vi "Autonomous.vi"() -> ()   [LabVIEW 2017]
doc: "This VI starts when autonomous period begins, and will automatically be terminated when it ends. You can carry out timed or sensor driven operations directly to I/O or to subsystems without needing to return to the caller."
uses:
  Shared/PathFileData.ctl
  Support Code/AutonomousRoutine.ctl
  b2a3c205-1cfd-49ae-9965-d89eaaa89800.vi
  <vilib>/Rock Robotics/WPI/Utilities/WPI_GetSetVariantRefNum.vi
  <vilib>/Rock Robotics/Network Tables/NT Read Boolean.vi
  <vilib>/Rock Robotics/Network Tables/NT Read Numeric Array.vi
  <vilib>/Rock Robotics/Network Tables/NT Read Number.vi
panel:
  out "PathData":T1
  out "File Path":string
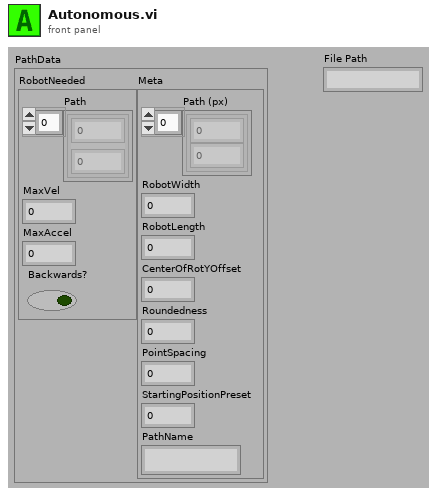
[diagram p1: front panel]
types:
  T1 = typedef "PathFileData.ctl" = cluster{"RobotNeeded":cluster{"Path":cluster{dbl, dbl}[], "MaxVel":dbl, "MaxAccel":dbl, "Backwards?":bool}, "Meta":cluster{"Path (px)":cluster{i32, i32}[], "RobotWidth":dbl, "RobotLength":dbl, "CenterOfRotYOffset":dbl, "Roundedness":dbl, "PointSpacing":dbl, "StartingPositionPreset":u32, "PathName":string}}
  T2 = typedef "AutonomousRoutine.ctl" = enum16{"Score Scale", "Score Switch"}
  T3 = typedef "WPI_JoystickDevRef.ctl" = cluster{"Device":T4}
  T4 = typedef "WPI_JoystickDeviceEnum.ctl" = enum16{"USB 0", "USB 1", "USB 2", "USB 3", "USB 4", "USB 5"}
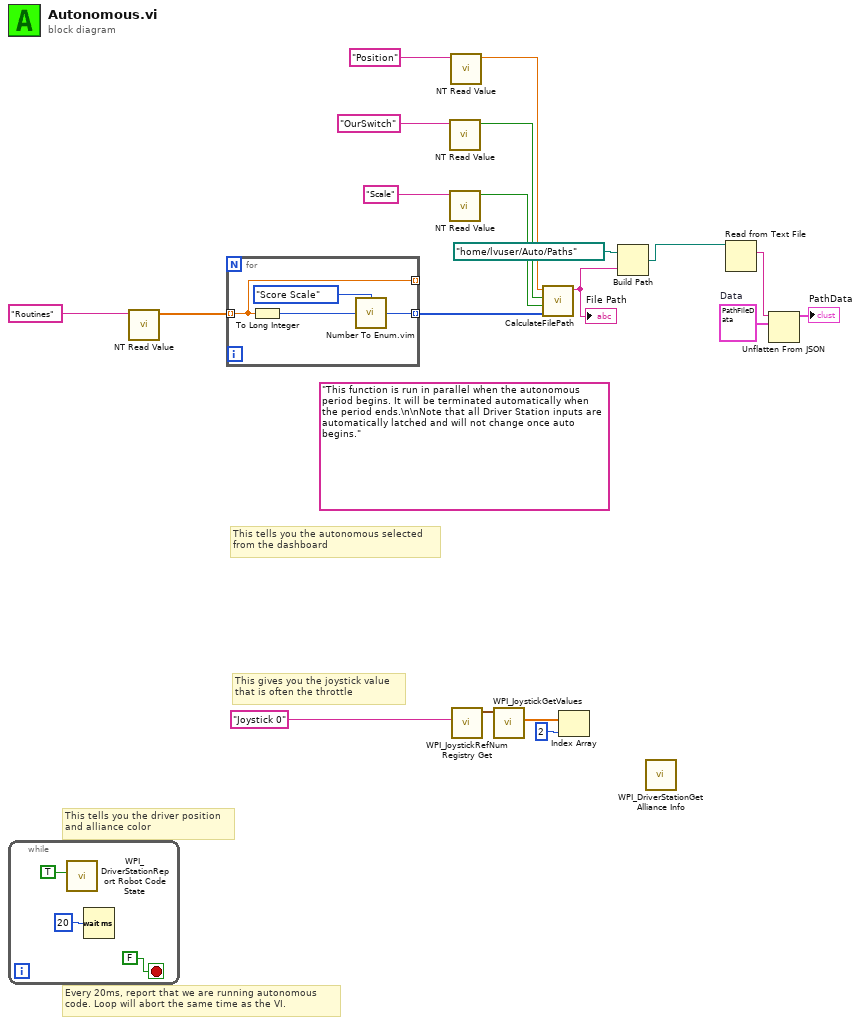
[diagram p0: block diagram]
diagram:
  w2 = T1 {"RobotNeeded"={"Path"=[], "MaxVel"=0.0, "MaxAccel"=0.0, "Backwards?"=FALSE}, "Meta"={"Path (px)"=[], "RobotWidth"=0.0, "RobotLength"=0.0, "CenterOfRotYOffset"=0.0, "Roundedness"=0.0, "PointSpacing"=0.0, "StartingPositionPreset"=0, "PathName"=""}}  # Data
  (unwired) "This function is run in parallel when the autonomous period begins. It will be terminated automatically when the period ends.\n\nNote that all Driver Station inputs are automatically latched and will not change once auto begins."
  # "This tells you the autonomous selected\nfrom the dashboard"
  # "Every 20ms, report that we are running autonomous\ncode. Loop will abort the same time as the VI."
  # "This gives you the joystick value\nthat is often the throttle"
  # "This tells you the driver position\nand alliance color"
  n1 = while {
    stop <- FALSE stop-if-true
    n2 = call <vilib>:"WPI_DriverStationReport Robot Code State.vi"("Autonomous"=TRUE) -> ()  [unwired: 10 in, 1 out]
    n3 = Wait (ms)(milliseconds to wait=u32 20) -> ()  [unwired: 1 out]
  }
  n4 = call-poly <vilib>:"NT Read Value.vi"("Name"="Routines") -> ("Numeric Array"=w11:dbl[])  [unwired: 9 in, 1 out]
  n5 = for {
    tunnel: w11 -> [w26] mode=indexing
    tunnel: [w26] -> _ mode=indexing
    tunnel: [w23] -> w7 mode=indexing
    n6 = To Long Integer(number=w26) -> (32bit integer=w25:i32)
    n7 = call "Number To Enum.vim"("number"=w25, "enum type"=AutonomousRoutine."Score Scale" ("LL")) -> ("number as enum"=w23:T2)
  }
  n8 = call-poly <vilib>:"NT Read Value.vi"("Name"="OurSwitch") -> ("Boolean"=w9:bool)  [unwired: 9 in, 1 out]
  n9 = call-poly <vilib>:"NT Read Value.vi"("Name"="Scale") -> ("Boolean"=w8:bool)  [unwired: 9 in, 1 out]
  n10 = call-poly <vilib>:"NT Read Value.vi"("Name"="Position") -> ("Numeric"=w10:dbl)  [unwired: 9 in, 1 out]
  n11 = call <vilib>:"WPI_JoystickRefNum Registry Get.vi"("refnum name"="Joystick 0") -> ("JoystickDevRef"=w18:T3)  [unwired: 1 in, 9 out]
  n12 = call <vilib>:"WPI_JoystickGetValues.vi"("JoystickDevRef"=w18) -> ("Axes"=w17:dbl[])  [unwired: 6 in, 4 out]
  n13 = call "CalculateFilePath.vi"("Routines"=w7, "Scale"=w8, "OurSwitch"=w9, "Position"=w10) -> ("File Name"=w6:string)  [unwired: 7 in]
  "File Path" <- w6
  n14 = Index Array(array=w17, index=2) -> ()  [unwired: 1 out]
  n15 = Build Path(base path=path "/home/lvuser/Auto/Paths", name or relative path=w6) -> (appended path=w4:path)
  n16 = call <vilib>:"WPI_DriverStationGet Alliance Info.vi"() -> ()  [unwired: 12 out]
  n17 = Read from Text File(file (use dialog)=w4) -> (text=w3:string)  [unwired: 3 in, 3 out]
  n18 = Unflatten From JSON(JSON string=w3, type and defaults=w2) -> (value=→"PathData":T1)  [unwired: 5 in, 1 out]
